vi "Initialize.vi"(5 "通讯设置 in":T1={"VISA resource name"="COM1", "Baud Rate"=19200, "Slave Address"=255}, 6 "Timeout":u32=1000) -> (0 "error out":errorcluster, 1 "Slave Address":u8, 2 "Timeout out":u32, 3 "VISA resource name out":refnum<visa-resource-name>, 4 "通讯设置 out":T1={"VISA resource name"="COM1", "Baud Rate"=19200, "Slave Address"=255})   [LabVIEW 2018]
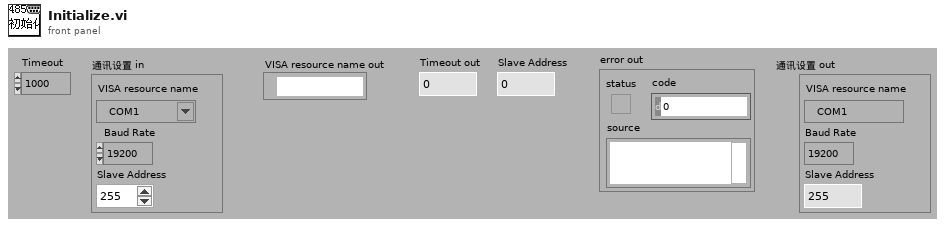
[diagram p1: front panel]
types:
  T1 = cluster{"VISA resource name":refnum<visa-resource-name>, "Baud Rate":u32, "Slave Address":u8}
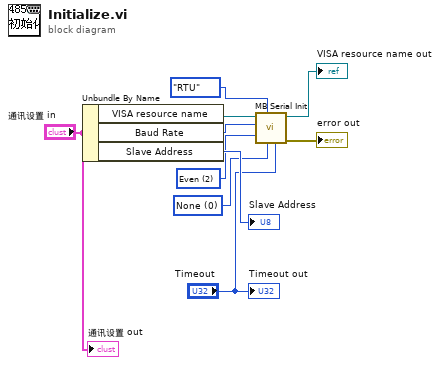
[diagram p0: block diagram]
diagram:
  w5 = u16 0 items=["None", "XON/XOFF", "RTS/CTS", "XON/XOFF & RTS/CTS", "DTR/DSR", "XON/XOFF & DTR/DSR"] ("Flow Control")
  w4 = u16 2 items=["None", "Odd", "Even", "Mark", "Space"] ("Parity")
  n1 = Unbundle By Name("通讯设置 in") -> ("VISA resource name"=w8:refnum<visa-resource-name>, "Baud Rate"=w9:u32, "Slave Address"=→"Slave Address":u8)
  n2 = call "MB Serial Init.vi"("Timeout"="Timeout", "Flow Control"=w5, "Mode"=enum16{"RTU", "ASCII"}."RTU", "Parity"=w4, "Baud Rate"=w9, "VISA resource name"=w8) -> ("error out"=→"error out":errorcluster, "VISA resource name out"=→"VISA resource name out":refnum<visa-resource-name>)  [unwired: 4 in]
  "通讯设置 out" <- "通讯设置 in"
  "Timeout out" <- "Timeout"
